vi "Read IC.lvclass.vi"(8 "error in (no error)":errorcluster, 11 "PDE.lvclass in":refnum<class "NI_PDE.lvclass">) -> (0 "error out":errorcluster, 2 "IC.lvclass":refnum<class "NI_IC.lvclass">[](array[class]), 3 "PDE.lvclass out":refnum<class "NI_PDE.lvclass">)   [LabVIEW 2020, in "NI_PDE.lvlib" / "NI_PDE.lvclass"]
uses:
  <vilib>/gmath/pde.llb/PDEClass/NI_PDE.lvclass
  <vilib>/gmath/pde.llb/ICClass/NI_IC.lvclass
  <vilib>/gmath/pde.llb/PDEClass/NI_PDE.lvclass/NI_PDE.ctl
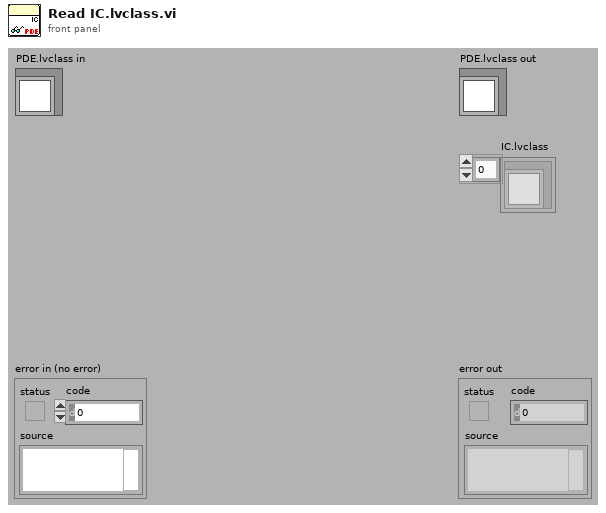
[diagram p1: front panel]
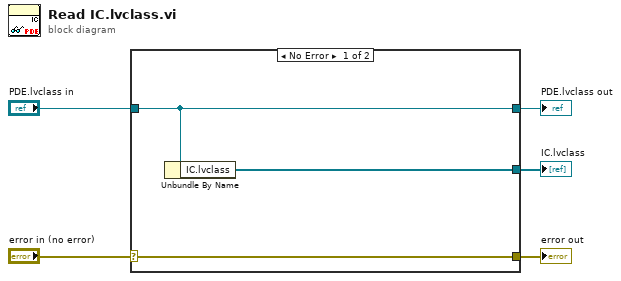
[diagram p0: block diagram]
diagram:
  n1 = case shown="No Error" "error in (no error)" {
    selector: "error in (no error)" -> [w8 w9]
    tunnel: [w8 w9] -> w4
    tunnel: [w7 w10] -> w2
    tunnel: "PDE.lvclass in" -> [w7 w10]
    tunnel: [w6 _] -> w1
    frame No Error {
      n2 = Unbundle By Name(w7) -> ("IC.lvclass"=w6:refnum<class "NI_IC.lvclass">[])
    }
    frame Error {
    }
  }
  "error out" <- w4
  "PDE.lvclass out" <- w2
  "IC.lvclass" <- w1
